vi "test_connection.vi"(0 "username@della.princeton.edu":string, 1 "password":string) -> (6 "Connection Successful":bool)   [LabVIEW 2019]
panel:
  out "standard error":string
  out "standard output":string
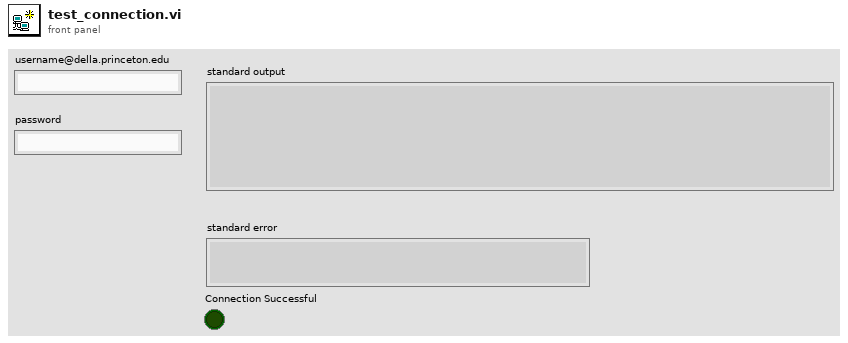
[diagram p1: front panel]
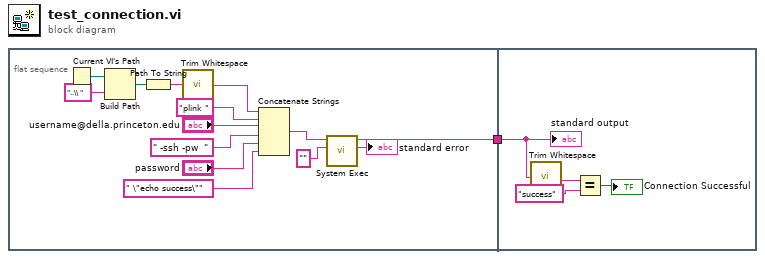
[diagram p0: block diagram]
diagram:
  n1 = flat-sequence {
    tunnel: [w5] -> w1
    tunnel: w1 -> [w18]
    frame #0 {
      n2 = Current VI's Path() -> (path=w11:path)
      n3 = Build Path(base path=w11, name or relative path="..\\ ") -> (appended path=w13:path)
      n4 = Path To String(path=w13) -> (string=w14:string)
      n5 = call <vilib>:"Trim Whitespace.vi"("string"=w14) -> ("trimmed string"=w15:string)  [unwired: 1 in]
      n6 = Concatenate Strings(w15, "plink ", "username@della.princeton.edu", " -ssh -pw  ", "password", " \"echo success\"") -> (w8:string)
      n7 = call <vilib>:"System Exec.vi"("standard input"="", "command line"=w8) -> ("standard error"=→"standard error":string, "standard output"=w5:string)  [unwired: 6 in, 2 out]
    }
    frame #1 {
      n8 = call <vilib>:"Trim Whitespace.vi"("string"=w18) -> ("trimmed string"=w19:string)  [unwired: 1 in]
      n9 = Equal?(x=w19, y="success") -> (x = y?=→"Connection Successful":bool)
      "standard output" <- w18
    }
  }
